vi "Capture Intruder.vi"(7 "File Path":path=path "C:/Users/jmart/OneDrive/Documents/College assignments/UCSD/ECE 144/Intruder.png", 8 "error in":errorcluster, 11 "Session In":T1) -> (0 "error out":errorcluster, 1 "Image":T2(plugin-control), 3 "Session Out":T1, 5 "File Path":path=path "C:/Users/jmart/OneDrive/Documents/College assignments/UCSD/ECE 144/Intruder.png")   [LabVIEW 2020]
doc: "Take a quick picture and save it in the File Path specified."
uses:
  <vilib>/userdefined/High Color/IMAQdx.ctl
  <vilib>/vision/driver/NI_Vision_Acquisition_Software.lvlib
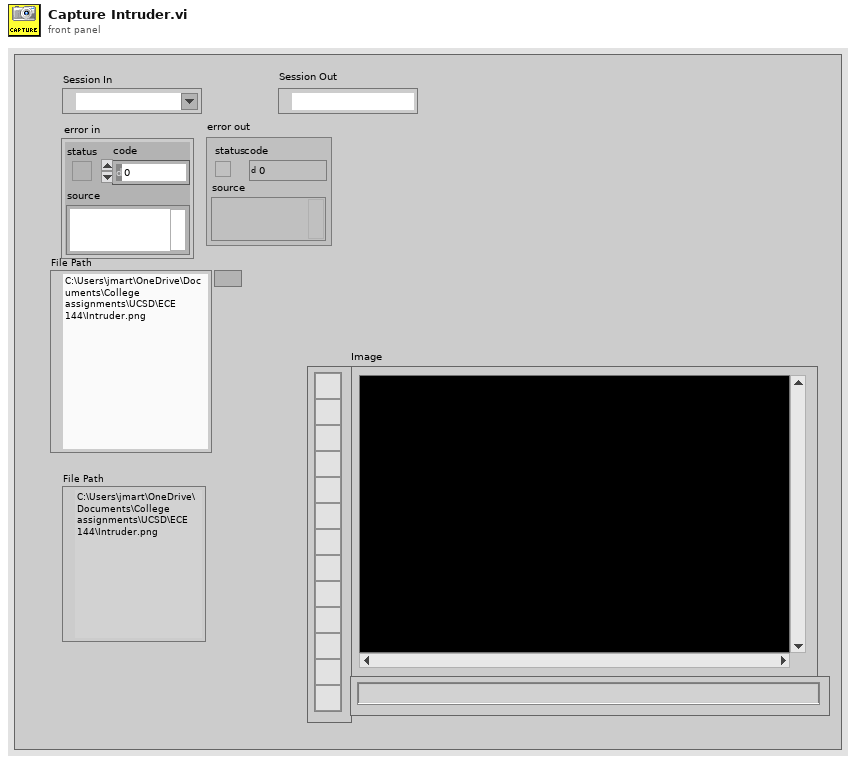
[diagram p1: front panel]
types:
  T1 = typedef "IMAQdx.ctl" = refnum<k21>
  T2 = typedef "IMAQ Image.ctl" = refnum<image>
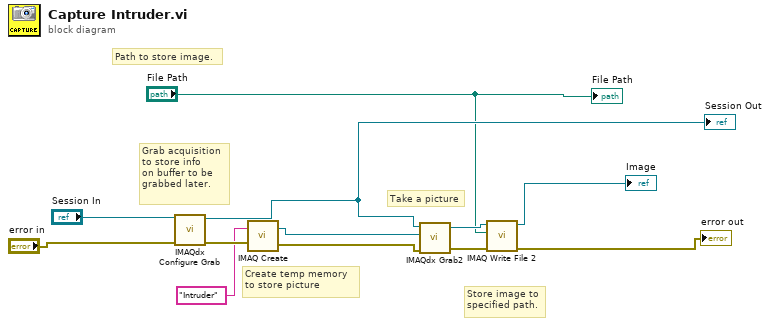
[diagram p0: block diagram]
diagram:
  # "Path to store image."
  # "Store image to\nspecified path."
  # "Take a picture"
  # "Create temp memory\nto store picture"
  # "Grab acquisition\nto store info\non buffer to be\ngrabbed later."
  n1 = call <vilib>:"IMAQdx Configure Grab.vi"("error in"="error in", "Session In"="Session In") -> ("error out"=w12:errorcluster, "Session Out"=w6:T1)  [unwired: 8 in]
  "Session Out" <- w6
  n2 = call "IMAQ Create"("Image Name"="Intruder", "error in (no error)"=w12) -> ("New Image"=w10:T2, "error out"=w9:errorcluster)  [unwired: 3 in]
  n3 = call <vilib>:"IMAQdx Grab2.vi"("error in"=w9, "Image In"=w10, "Session In"=w6) -> ("error out"=w7:errorcluster, "Image Out"=w8:T2)  [unwired: 5 in, 2 out]
  n4 = call-poly "IMAQ Write File 2"("error in (no error)"=w7, "File Path"="File Path", "Image"=w8) -> ("error out"=→"error out":errorcluster, "Image Out (duplicate)"=→"Image":T2)  [unwired: 7 in]
  "File Path" <- "File Path"
